vi "Code 0.0.1.vi"() -> ()   [LabVIEW 2017]
uses:
  <vilib>/Instr/_visa.llb/VISA Configure Serial Port (Instr).vi
panel:
  in  "Flash Baudrate":u32(ring)=230400 items=["4800"=4800, "9600"=9600, "19200"=19200, "38400"=38400, "57600"=57600, "115200"=115200, "230400"=230400, "460800"=460800, "921600"=921600]
  in  "cmd Baudrate":u32(ring)=230400 items=["4800"=4800, "9600"=9600, "19200"=19200, "38400"=38400, "57600"=57600, "115200"=115200, "230400"=230400, "460800"=460800, "921600"=921600]
  in  "UUT COM Port":refnum<visa-resource-name>="COM4"
  in  "Next Button":bool
  in  "File Path Control":path
  out "Status":bool
  out "cmd Sent":bool
  out "CheckSumArray":u16[][](array[numeric]) format="%.0x"
  out "CheckSum":bool[][](array[boolean])
  in  "stop 9":bool
  in  "stop 8":bool
  out "CheckSum DataB":u16 format="%.0x"
  out "CheckSum Data":u16 format="%.0x"
  in  "stop 5":bool
  in  "stop 4":bool
  out "Array 3":u16[][](array[numeric]) format="%.0x"
  out "Num of Data packet":i32
  out "Writting Data":bool
  out "Size of Text File":i32
  out "Full Text File":u8[](array[numeric]) format="%.0x"
  out "All bytes in file in HEX U8":u8[](array[numeric]) format="%02x"
  out "Send Header":bool
  out "AutoBaud Success":bool
  out "sumHeader":u16 format="%.0x"
  in  "stop 3":bool
  in  "stop 2":bool
  out "error out":errorcluster
  in  "stop":bool
  out "Autobaud":string
  # "Ver 0.0.1"
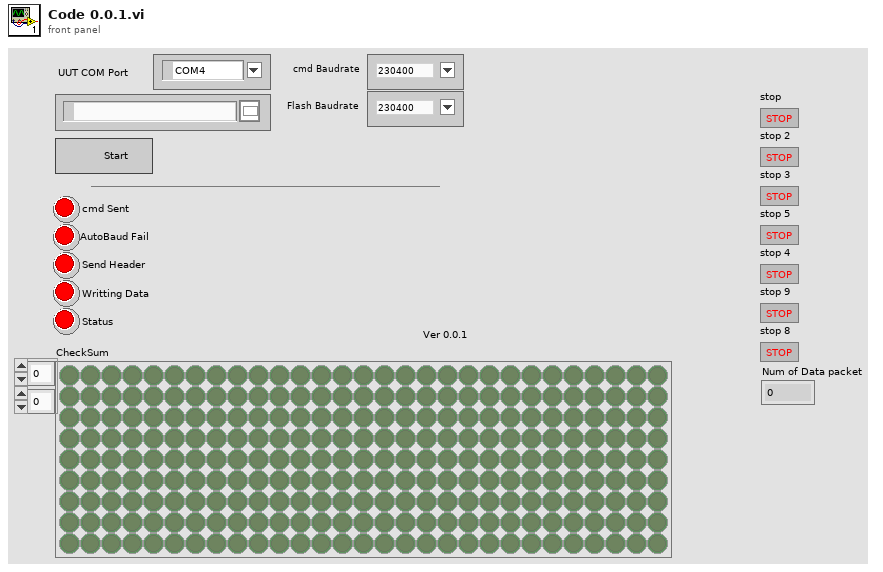
[diagram p1: front panel]
types:
  T1 = enum16{"open", "replace", "create", "open or create", "replace or create", "replace or create with confirmation"}
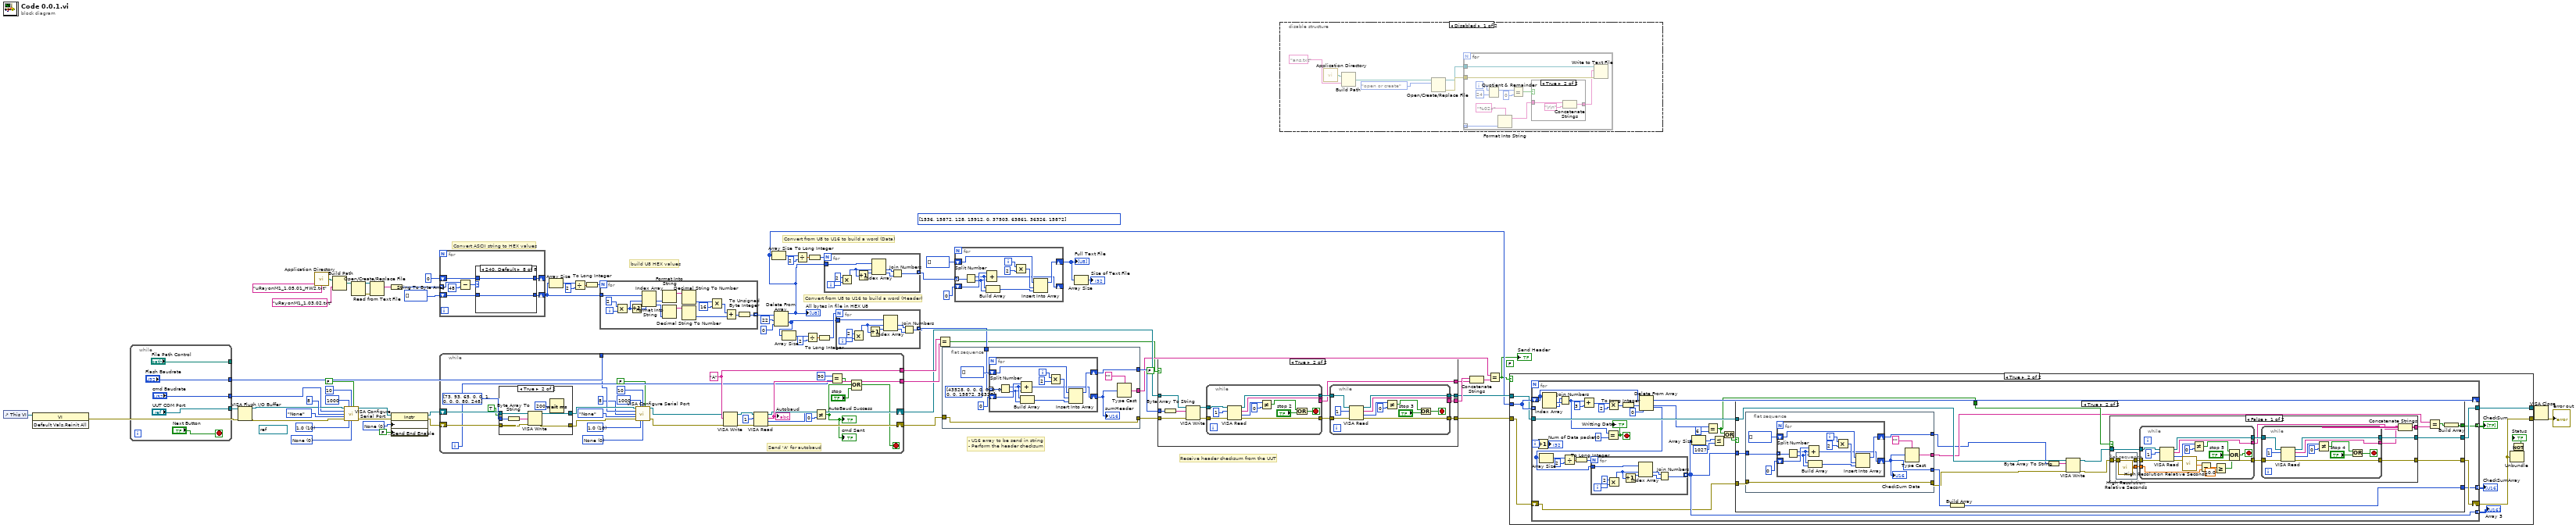
[diagram p0: block diagram]
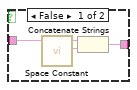
[diagram p3: hidden frame]
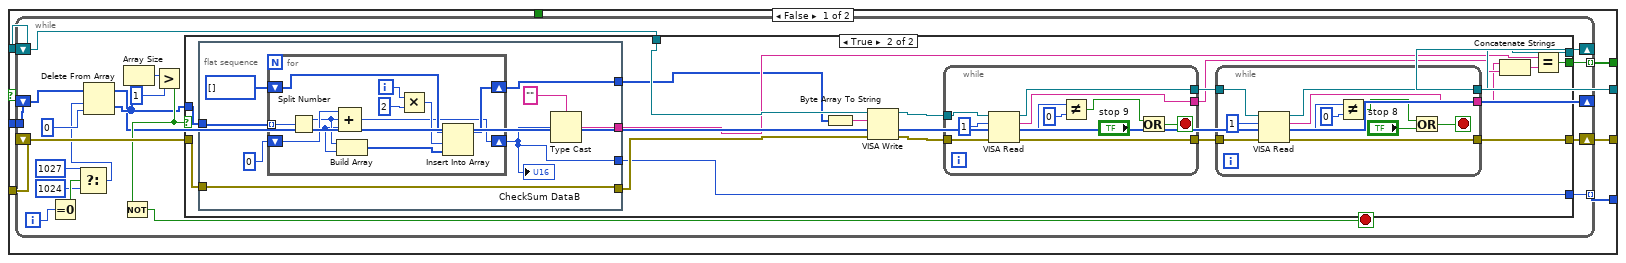
[diagram p6: hidden frame]
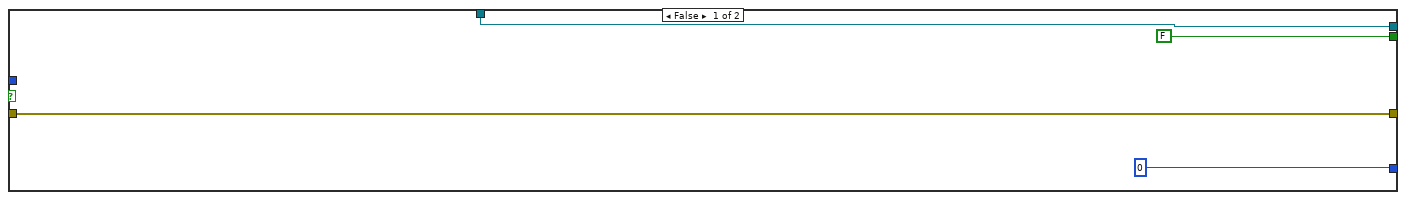
[diagram p7: hidden frame]
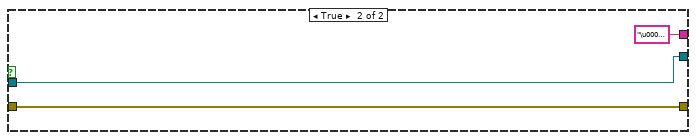
[diagram p8: hidden frame]
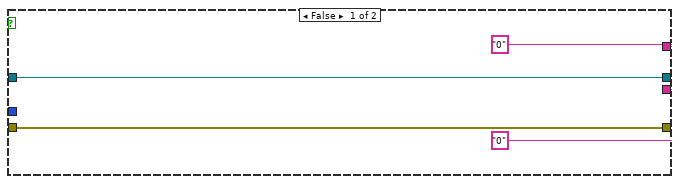
[diagram p9: hidden frame]
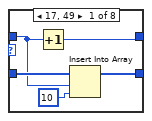
[diagram p10: hidden frame]
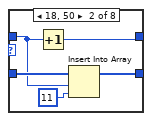
[diagram p11: hidden frame]
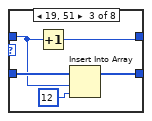
[diagram p12: hidden frame]
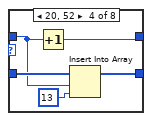
[diagram p13: hidden frame]
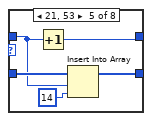
[diagram p14: hidden frame]
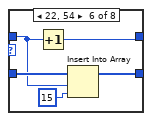
[diagram p15: hidden frame]
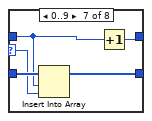
[diagram p16: hidden frame]
diagram:
  (unwired) FALSE
  (unwired) FALSE
  (unwired) u16[] [1536, 15872, 128, 15912, 0, 37503, 63861, 36326, 15872] ("Array 4")
  (unwired) refnum<visa-resource-name> "COM4" ("VISA resource name")
  w32 = u16 0 items=["None", "LastBit", "TermChar", "Break"] ("Serial Settings:Serial End Mode for Writes")
  w36 = u16 0 items=["None", "XON/XOFF", "RTS/CTS", "XON/XOFF & RTS/CTS", "DTR/DSR", "XON/XOFF & DTR/DSR"] ("flow control (0:none)")
  w37 = u16 10 items=["1.0"=10, "1.5"=15, "2.0"=20] ("stop bits (10: 1 bit)")
  (unwired) "uRayonM1_1.05.01_HW2.txt" ("name or relative path")
  # "Receive header checksum from the UUT"
  # "- U16 array to be send in string\n- Perform the header checksum"
  # "Convert from U8 to U16 to build a word (Header)"
  # "build U8 HEX values"
  # "Convert from U8 to U16 to build a word (Data)"
  # "Convert ASCII string to HEX values"
  n1 = control-ref of="This VI"() -> (w8:refnum<vi>)
  n2 = invoke class="VI" method="Default Vals.Reinit All"(reference=w8) -> (error out=w11:errorcluster)  [unwired: 2 in, 2 out]
  n3 = while {
    tunnel: ["UUT COM Port"] -> w4
    tunnel: ["Flash Baudrate"] -> w3
    tunnel: ["cmd Baudrate"] -> w2
    tunnel: ["File Path Control"] -> _
    stop <- "Next Button" stop-if-true
  }
  n4 = VISA Flush I/O Buffer(VISA resource name=w4, error in (no error)=w11) -> (VISA resource name out=w9:refnum<visa-resource-name>, error out=w10:errorcluster)  [unwired: 1 in]
  n5 = call <vilib>:"Application Directory.vi"() -> ("Application Directory"=w63:path)
  n6 = Build Path(base path=w63, name or relative path="uRayonM1_1.03.02.txt") -> (appended path=w1:path)
  n7 = call-poly "VISA Configure Serial Port"("VISA resource name"=w9, "timeout (10sec)"=u32 1000, "termination char\n(0xA = '\\n' = LF)"=u8 10 ("termination char\n(0xA = '\\n' = LF)"), "Enable Termination\nChar (T)"=FALSE ("Enable Termination\nChar (T)"), "baud rate (9600)"=w2, "data bits (8)"=u16 8, "parity (0:none)"=enum16{"None", "Odd", "Even", "Mark", "Space"}."None", "error in (no error)"=w10, "stop bits (10: 1 bit)"=w37, "flow control (0:none)"=w36) -> ("VISA resource name out"=w34:refnum<visa-resource-name>, "error out"=w35:errorcluster)  [unwired: 4 in]
  n8 = Open/Create/Replace File(file path (use dialog)=w1) -> (refnum out=w61:refnum<file>, error out=w62:errorcluster)  [unwired: 5 in, 1 out]
  n9 = Read from Text File(file (use dialog)=w61, error in=w62) -> (text=w59:string)  [unwired: 2 in, 3 out]
  n10 = String To Byte Array(string=w59) -> (unsigned byte array=w60:u8[])
  n11 = property class="Instr"(reference=w34, error in=w35, "Serial Settings:End Mode for Writes"=w32, "Message Based Settings:Send End Enable"=FALSE) -> (reference out=w7:refnum<visa-resource-name>, error out=w6:errorcluster)
  n12 = for {
    tunnel: w60 -> [w82] mode=indexing
    shift-right: [w78] -> w56
    shift-left: u8[] [] -> [w79]
    shift-right: [w77] -> _
    shift-left: 0 ("y") -> [w76]
    n13 = Subtract(x=w82, y=u8 48) -> (x-y=w80:u8)
    n14 = case shown="240, Default" w80 {
      selector: w80 -> [_ _ _ _ _ _ w116 _]
      tunnel: [w85 w90 w96 w100 w105 w110 w115 w119] -> w78
      tunnel: w79 -> [w87 w91 w97 w102 w107 w112 w117 w119]
      tunnel: [w83 w88 w93 w98 w103 w108 w113 w118] -> w77
      tunnel: w76 -> [w84 w89 w94 w99 w104 w109 w114 w118]
      frame 17, 49 {
        n15 = Increment(x=w84) -> (x+1=w83:i32)
        n16 = Insert Into Array(array=w87, index=w84, new element=u8 10) -> (w85:u8[])
      }
      frame 18, 50 {
        n17 = Increment(x=w89) -> (x+1=w88:i32)
        n18 = Insert Into Array(array=w91, index=w89, new element=u8 11) -> (w90:u8[])
      }
      frame 19, 51 {
        n19 = Increment(x=w94) -> (x+1=w93:i32)
        n20 = Insert Into Array(array=w97, index=w94, new element=u8 12) -> (w96:u8[])
      }
      frame 20, 52 {
        n21 = Increment(x=w99) -> (x+1=w98:i32)
        n22 = Insert Into Array(array=w102, index=w99, new element=u8 13) -> (w100:u8[])
      }
      frame 21, 53 {
        n23 = Increment(x=w104) -> (x+1=w103:i32)
        n24 = Insert Into Array(array=w107, index=w104, new element=u8 14) -> (w105:u8[])
      }
      frame 22, 54 {
        n25 = Increment(x=w109) -> (x+1=w108:i32)
        n26 = Insert Into Array(array=w112, index=w109, new element=u8 15) -> (w110:u8[])
      }
      frame 0..9 {
        n27 = Insert Into Array(array=w117, index=w114, new element=w116) -> (w115:u8[])
        n28 = Increment(x=w114) -> (x+1=w113:i32)
      }
      frame 240, Default {
      }
    }
  }
  n29 = while {
    tunnel: [w150] -> w70
    tunnel: [w149] -> w69
    shift-right: [w148] -> w68
    shift-left: w7 -> [w146]
    shift-right: [w147] -> w66
    shift-left: w6 -> [w145]
    tunnel: w3 -> [w127]
    i -> [w133]
    stop <- w136 stop-if-true
    w120 = u16 0 items=["None", "XON/XOFF", "RTS/CTS", "XON/XOFF & RTS/CTS", "DTR/DSR", "XON/XOFF & DTR/DSR"] ("flow control (0:none)")
    w121 = u16 10 items=["1.0"=10, "1.5"=15, "2.0"=20] ("stop bits (10: 1 bit)")
    w149 = "A" ("write buffer")
    # "Send 'A' for autobaud"
    n30 = case shown="True" TRUE {
      tunnel: w146 -> [w152 w159]
      tunnel: w145 -> [w151 w158]
      tunnel: [w152 w157] -> w128
      tunnel: [w151 w156] -> w129
      tunnel: u8[] [73, 93, 65, 0, 0, 1, 0, 0, 0, 80, 248] ("output array") -> [_ w155]
      frame False {
      }
      frame True {
        n31 = Byte Array To String(unsigned byte array=w155) -> (string=w154:string)
        n32 = VISA Write(VISA resource name=w159, write buffer=w154, error in (no error)=w158) -> (VISA resource name out=w157:refnum<visa-resource-name>, error out=w156:errorcluster)  [unwired: 1 out]
        n33 = Wait (ms)(milliseconds to wait=u32 200) -> ()  [unwired: 1 out]
      }
    }
    n34 = call-poly "VISA Configure Serial Port"("VISA resource name"=w128, "timeout (10sec)"=u32 1000, "termination char\n(0xA = '\\n' = LF)"=u8 10 ("termination char\n(0xA = '\\n' = LF)"), "Enable Termination\nChar (T)"=FALSE ("Enable Termination\nChar (T)"), "baud rate (9600)"=w127, "data bits (8)"=u16 8, "parity (0:none)"=enum16{"None", "Odd", "Even", "Mark", "Space"}."None", "error in (no error)"=w129, "stop bits (10: 1 bit)"=w121, "flow control (0:none)"=w120) -> ("VISA resource name out"=w130:refnum<visa-resource-name>, "error out"=w131:errorcluster)  [unwired: 4 in]
    n35 = VISA Write(VISA resource name=w130, write buffer=w149, error in (no error)=w131) -> (VISA resource name out=w139:refnum<visa-resource-name>, error out=w138:errorcluster)  [unwired: 1 out]
    n36 = VISA Read(VISA resource name=w139, byte count=u32 1, error in (no error)=w138) -> (VISA resource name out=w148:refnum<visa-resource-name>, read buffer=w150:string, return count=w141:u32, error out=w147:errorcluster)
    "Autobaud" <- w150
    n37 = Not Equal?(x=w141, y=u32 0) -> (x != y?=w132:bool)
    "AutoBaud Success" <- w132
    "cmd Sent" <- w132
    n38 = Equal?(x=90, y=w133) -> (x = y?=w134:bool)
    n39 = Compound Arithmetic op=OR(w134, w132, "stop") -> (w136:bool)
  }
  n40 = Array Size(array=w56) -> (size(s)=w55:i32)
  n41 = Divide(x=w55, y=2) -> (x/y=w53:dbl)
  n42 = To Long Integer(number=w53) -> (32bit integer=w52:i32)
  n43 = for {
    N: w52 -> [_]
    tunnel: w56 -> [w174]
    tunnel: [w160] -> w51 mode=indexing
    i -> [w173]
    n44 = Multiply(x=2, y=w173) -> (x*y=w171:i32)
    n45 = Increment(x=w171) -> (x+1=w170:i32)
    n46 = Index Array(array=w174, index #1=w171, index #2=w170) -> (element #1=w163:u8, element #2=w162:u8)
    n47 = Format Into String(w163) -> (resulting string=w164:string)  [unwired: 3 in, 1 out]
    n48 = Format Into String(w162) -> (resulting string=w169:string)  [unwired: 3 in, 1 out]
    n49 = Decimal String To Number(string=w164) -> (number=w165:i32)  [unwired: 2 in, 1 out]
    n50 = Decimal String To Number(string=w169) -> (number=w168:i32)  [unwired: 2 in, 1 out]
    n51 = Multiply(x=w165, y=16) -> (x*y=w167:i32)
    n52 = Add(x=w167, y=w168) -> (x+y=w161:i32)
    n53 = To Unsigned Byte Integer(number=w161) -> (unsigned 8bit integer=w160:u8)
  }
  n54 = Delete From Array(array=w51, length=22, index=0) -> (deleted portion=w22:u8[], array with subset deleted=w14:u8[])
  "All bytes in file in HEX U8" <- w14
  n55 = Array Size(array=w14) -> (size(s)=w28:i32)
  n56 = Array Size(array=w22) -> (size(s)=w27:i32)
  n57 = Divide(x=w28, y=2) -> (x/y=w30:dbl)
  n58 = Divide(x=w27, y=2) -> (x/y=w25:dbl)
  n59 = To Long Integer(number=w30) -> (32bit integer=w23:i32)
  n60 = To Long Integer(number=w25) -> (32bit integer=w24:i32)
  n61 = for {
    N: w23 -> [_]
    tunnel: w14 -> [w179]
    tunnel: [w175] -> w15 mode=indexing
    i -> [w178]
    n62 = Multiply(x=2, y=w178) -> (x*y=w181:i32)
    n63 = Increment(x=w181) -> (x+1=w182:i32)
    n64 = Index Array(array=w179, index #1=w181, index #2=w182) -> (element #1=w177:u8, element #2=w176:u8)
    n65 = Join Numbers(hi=w177, lo=w176) -> ((hi.lo)=w175:u16)
  }
  n66 = for {
    N: w24 -> [_]
    tunnel: w22 -> [w187]
    tunnel: [w183] -> w21 mode=indexing
    i -> [w186]
    n67 = Multiply(x=2, y=w186) -> (x*y=w189:i32)
    n68 = Increment(x=w189) -> (x+1=w190:i32)
    n69 = Index Array(array=w187, index #1=w189, index #2=w190) -> (element #1=w185:u8, element #2=w184:u8)
    n70 = Join Numbers(hi=w185, lo=w184) -> ((hi.lo)=w183:u16)
  }
  n71 = Equal?(x=w69, y=w70) -> (x = y?=w12:bool)
  n72 = flat-sequence {
    tunnel: w66 -> [w191]
    tunnel: [w196] -> w65
    tunnel: [w193] -> w64
    tunnel: w21 -> [w192]
    tunnel: [w191] -> w20
    frame #0 {
      (unwired) u16[] [43528, 0, 0, 0, 0, 0, 0, 0, 0, 15872, 36326]
      n73 = for {
        tunnel: w192 -> [w209] mode=indexing
        shift-right: [w204] -> w196
        shift-left: u8[] [] -> [w203]
        shift-right: [w201] -> w195
        shift-left: u16 0 -> [w202]
        i -> [w208]
        n74 = Split Number(x=w209) -> (hi(x)=w200:u8, lo(x)=w199:u8)
        n75 = Build Array(w200, w199) -> (w206:u8[])
        n76 = Compound Arithmetic op=ADD(w202, w200, w199) -> (w201:u16)
        n77 = Multiply(x=w208, y=2) -> (x*y=w205:i32)
        n78 = Insert Into Array(array=w203, index=w205, new element=w206) -> (w204:u8[])
      }
      "sumHeader" <- w195
      n79 = Type Cast(type="", x=w195) -> (*(type *) &x=w193:string)
    }
  }
  n80 = for {
    tunnel: w15 -> [w220] mode=indexing
    shift-right: [w215] -> w17
    shift-left: u8[] [] -> [w214]
    shift-right: [w212] -> _
    shift-left: u16 0 -> [w213]
    i -> [w219]
    n81 = Split Number(x=w220) -> (hi(x)=w211:u8, lo(x)=w210:u8)
    n82 = Build Array(w211, w210) -> (w217:u8[])
    n83 = Compound Arithmetic op=ADD(w213, w211, w210) -> (w212:u16)
    n84 = Multiply(x=w219, y=2) -> (x*y=w216:i32)
    n85 = Insert Into Array(array=w214, index=w216, new element=w217) -> (w215:u8[])
  }
  "Full Text File" <- w17
  n86 = Array Size(array=w17) -> (size(s)=→"Size of Text File":i32)
  n87 = case shown="True" w12 {
    tunnel: w20 -> [w223 w232]
    tunnel: w68 -> [w224 w231]
    tunnel: [w223 w230] -> w42
    tunnel: [w224 w229] -> w43
    tunnel: w65 -> [_ w228]
    tunnel: ["0" ("read buffer") w227] -> w46
    tunnel: ["0" ("read buffer") w226] -> w45
    frame False {
    }
    frame True {
      n88 = Byte Array To String(unsigned byte array=w228) -> (string=w225:string)
      n89 = VISA Write(VISA resource name=w231, write buffer=w225, error in (no error)=w232) -> (VISA resource name out=w234:refnum<visa-resource-name>, error out=w233:errorcluster)  [unwired: 1 out]
      n90 = while {
        tunnel: w234 -> [w255]
        tunnel: [w256] -> w235
        tunnel: w233 -> [w254]
        tunnel: [w257] -> w236
        tunnel: [w248] -> w226
        stop <- w250 stop-if-true
        n91 = VISA Read(VISA resource name=w255, byte count=u32 1, error in (no error)=w254) -> (VISA resource name out=w256:refnum<visa-resource-name>, read buffer=w248:string, return count=w249:u32, error out=w257:errorcluster)
        n92 = Not Equal?(x=w249, y=u32 0) -> (x != y?=w252:bool)
        n93 = Or(x=w252, y="stop 2") -> (x .or. y?=w250:bool)
      }
      n94 = while {
        tunnel: w235 -> [w246]
        tunnel: [w243] -> w229
        tunnel: w236 -> [w247]
        tunnel: [w244] -> w230
        tunnel: [w237] -> w227
        stop <- w238 stop-if-true
        n95 = VISA Read(VISA resource name=w246, byte count=u32 1, error in (no error)=w247) -> (VISA resource name out=w243:refnum<visa-resource-name>, read buffer=w237:string, return count=w239:u32, error out=w244:errorcluster)
        n96 = Not Equal?(x=w239, y=u32 0) -> (x != y?=w242:bool)
        n97 = Or(x=w242, y="stop 3") -> (x .or. y?=w238:bool)
      }
    }
  }
  n98 = disable-structure shown="Disabled" {
    frame Disabled {
      n99 = call <vilib>:"Application Directory.vi"() -> ("Application Directory"=w263:path)
      n100 = Build Path(base path=w263, name or relative path="ans.txt") -> (appended path=w262:path)
      n101 = Open/Create/Replace File(file path (use dialog)=w262, operation (0:open)=T1."open or create") -> (refnum out=w259:refnum<file>, error out=w260:errorcluster)  [unwired: 4 in, 1 out]
      n102 = for {
        tunnel: _ -> [w275] mode=indexing
        tunnel: w260 -> [w273]
        tunnel: w259 -> [w272]
        i -> [w268]
        n103 = Quotient & Remainder(x=w268, y=24 ("x")) -> (x-y*floor(x/y)=w266:i32)  [unwired: 1 out]
        n104 = Format Into String(format string="%02x", w275) -> (resulting string=w271:string)  [unwired: 2 in, 1 out]
        n105 = Equal?(x=w266, y=0) -> (x = y?=w269:bool)
        n106 = case shown="True" w269 {
          tunnel: w271 -> [w278 w281]
          tunnel: [w277 w280] -> w270
          frame False {
            n107 = call <vilib>:"Space Constant.vi"() -> ("String"=w276:string)
            n108 = Concatenate Strings(w278, w276) -> (w277:string)
          }
          frame True {
            n109 = Concatenate Strings(w281, "\r\n") -> (w280:string)
          }
        }
        n110 = Write to Text File(file (use dialog)=w272, text=w270, error in=w273) -> ()  [unwired: 1 in, 3 out]
      }
    }
    frame Enabled {
    }
  }
  n111 = Concatenate Strings(w46, w45) -> (w44:string)
  n112 = Equal?(x=w64, y=w44) -> (x = y?=w13:bool)
  "Send Header" <- w13
  n113 = case shown="True" w13 {
    tunnel: w43 -> [w283 w291]
    tunnel: w42 -> [w282 w287]
    tunnel: [w283 w290] -> w48
    tunnel: [w282 w286] -> w47
    tunnel: w14 -> [_ w292]
    frame False {
    }
    frame True {
      n114 = for {
        shift-right: [w315] -> _
        shift-left: w292 -> [w326]
        tunnel: w292 -> [_] mode=indexing
        tunnel: [w308] -> w293 mode=indexing
        tunnel: w291 -> [w307]
        tunnel: [w303] -> w290
        tunnel: [w301] -> w289 mode=indexing
        tunnel: [w300] -> w288 mode=indexing
        shift-right: [w302] -> w286
        shift-left: w287 -> [w294]
        i -> [w316]
        stop <- w319 stop-if-true
        n115 = Increment(x=w316) -> (x+1=→"Num of Data packet":i32)
        n116 = Index Array(array=w326) -> (element #1=w325:u8, element #2=w324:u8)  [unwired: 2 in]
        n117 = Join Numbers(hi=w324, lo=w325) -> ((hi.lo)=w296:u16)
        n118 = Add(x=w296, y=u32 3) -> (x+y=w322:u32)
        n119 = Equal?(x=w296, y=u16 0) -> (x = y?=w319:bool)
        "Writting Data" <- w319
        n120 = Multiply(x=w322, y=u32 2) -> (x*y=w320:u32)
        n121 = To Long Integer(number=w320) -> (32bit integer=w297:i32)
        n122 = Delete From Array(array=w326, length=w297, index=0) -> (deleted portion=w298:u8[], array with subset deleted=w315:u8[])
        n123 = Array Size(array=w298) -> (size(s)=w312:i32)
        n124 = Divide(x=w312, y=2) -> (x/y=w314:dbl)
        n125 = To Long Integer(number=w314) -> (32bit integer=w311:i32)
        n126 = for {
          N: w311 -> [_]
          tunnel: w298 -> [w499]
          tunnel: [w495] -> w308 mode=indexing
          i -> [w498]
          n127 = Multiply(x=2, y=w498) -> (x*y=w501:i32)
          n128 = Increment(x=w501) -> (x+1=w502:i32)
          n129 = Index Array(array=w499, index #1=w501, index #2=w502) -> (element #1=w497:u8, element #2=w496:u8)
          n130 = Join Numbers(hi=w497, lo=w496) -> ((hi.lo)=w495:u16)
        }
        n131 = Array Size(array=w308) -> (size(s)=w310:i32)
        n132 = Equal?(x=w297, y=6) -> (x = y?=w295:bool)
        n133 = Less Or Equal?(x=w310, y=1027) -> (x <= y?=w305:bool)
        n134 = Or(x=w295, y=w305) -> (x .or. y?=w304:bool)
        n135 = case shown="True" w304 {
          tunnel: w294 -> [w330 w429]
          tunnel: w307 -> [w333 w420]
          tunnel: [w332 w432] -> w302
          tunnel: [w331 w431] -> w303
          tunnel: w308 -> [w328 w430]
          tunnel: [w329 w426] -> w301
          tunnel: [w327 w424] -> w300
          tunnel: w295 -> [_ w423]
          frame False {
            n136 = while {
              tunnel: w328 -> [_]
              tunnel: [w348] -> w329 mode=indexing
              shift-right: [w350] -> w331
              shift-left: w333 -> [w352]
              shift-right: [w351] -> w332
              shift-left: w330 -> [w349]
              shift-right: [w340] -> _
              shift-left: w328 -> [w347]
              tunnel: [w339] -> w327 mode=indexing
              i -> [w338]
              stop <- w342 stop-if-true
              n137 = Equal To 0?(x=w338) -> (x = 0?=w337:bool)
              n138 = Select(t=1027 ("length"), s=w337, f=1024 ("length")) -> (s? t:f=w334:i32)
              n139 = Delete From Array(array=w347, length=w334, index=0) -> (deleted portion=w341:u16[], array with subset deleted=w340:u16[])
              n140 = Array Size(array=w341) -> (size(s)=w345:i32)
              n141 = Greater?(x=w345, y=1) -> (0:w343:bool)
              n142 = Not(x=w343) -> (.not. x?=w342:bool)
              n143 = case shown="True" w343 {
                tunnel: w352 -> [w354 w370]
                tunnel: [w356 w369] -> w351
                tunnel: [w354 w368] -> w350
                tunnel: w349 -> [w356 w366]
                tunnel: [FALSE w361] -> w348
                tunnel: w341 -> [_ w360]
                tunnel: [u16 0 ("Numeric") w359] -> w339
                frame False {
                }
                frame True {
                  n144 = flat-sequence {
                    tunnel: w366 -> [w376]
                    tunnel: [w380] -> w357
                    tunnel: [w378] -> w362
                    tunnel: w360 -> [w377]
                    tunnel: [w376] -> w367
                    tunnel: [w375] -> w359
                    frame #0 {
                      n145 = for {
                        tunnel: w377 -> [w393] mode=indexing
                        shift-right: [w388] -> w380
                        shift-left: u8[] [] -> [w387]
                        shift-right: [w385] -> w375
                        shift-left: u16 0 -> [w386]
                        i -> [w392]
                        n146 = Split Number(x=w393) -> (hi(x)=w384:u8, lo(x)=w383:u8)
                        n147 = Build Array(w384, w383) -> (w390:u8[])
                        n148 = Compound Arithmetic op=ADD(w386, w384, w383) -> (w385:u16)
                        n149 = Multiply(x=w392, y=2) -> (x*y=w389:i32)
                        n150 = Insert Into Array(array=w387, index=w389, new element=w390) -> (w388:u8[])
                      }
                      "CheckSum DataB" <- w375
                      n151 = Type Cast(type="", x=w375) -> (*(type *) &x=w378:string)
                    }
                  }
                  n152 = Byte Array To String(unsigned byte array=w357) -> (string=w358:string)
                  n153 = VISA Write(VISA resource name=w370, write buffer=w358, error in (no error)=w367) -> (VISA resource name out=w372:refnum<visa-resource-name>, error out=w371:errorcluster)  [unwired: 1 out]
                  n154 = while {
                    tunnel: w372 -> [w412]
                    tunnel: [w413] -> w373
                    tunnel: w371 -> [w411]
                    tunnel: [w414] -> w374
                    tunnel: [w405] -> w365
                    stop <- w407 stop-if-true
                    n155 = VISA Read(VISA resource name=w412, byte count=u32 1, error in (no error)=w411) -> (VISA resource name out=w413:refnum<visa-resource-name>, read buffer=w405:string, return count=w406:u32, error out=w414:errorcluster)
                    n156 = Not Equal?(x=w406, y=u32 0) -> (x != y?=w409:bool)
                    n157 = Or(x=w409, y="stop 9") -> (x .or. y?=w407:bool)
                  }
                  n158 = while {
                    tunnel: w373 -> [w403]
                    tunnel: [w400] -> w368
                    tunnel: w374 -> [w404]
                    tunnel: [w401] -> w369
                    tunnel: [w394] -> w364
                    stop <- w395 stop-if-true
                    n159 = VISA Read(VISA resource name=w403, byte count=u32 1, error in (no error)=w404) -> (VISA resource name out=w400:refnum<visa-resource-name>, read buffer=w394:string, return count=w396:u32, error out=w401:errorcluster)
                    n160 = Not Equal?(x=w396, y=u32 0) -> (x != y?=w399:bool)
                    n161 = Or(x=w399, y="stop 8") -> (x .or. y?=w395:bool)
                  }
                  n162 = Concatenate Strings(w364, w365) -> (w363:string)
                  n163 = Equal?(x=w362, y=w363) -> (x = y?=w361:bool)
                }
              }
            }
          }
          frame True {
            n164 = flat-sequence {
              tunnel: w429 -> [w477]
              tunnel: [w481] -> w416
              tunnel: [w479] -> w418
              tunnel: w430 -> [w478]
              tunnel: [w477] -> w419
              tunnel: [w476] -> w425
              frame #0 {
                n165 = for {
                  tunnel: w478 -> [w494] mode=indexing
                  shift-right: [w489] -> w481
                  shift-left: u8[] [] -> [w488]
                  shift-right: [w486] -> w476
                  shift-left: u16 0 -> [w487]
                  i -> [w493]
                  n166 = Split Number(x=w494) -> (hi(x)=w485:u8, lo(x)=w484:u8)
                  n167 = Build Array(w485, w484) -> (w491:u8[])
                  n168 = Compound Arithmetic op=ADD(w487, w485, w484) -> (w486:u16)
                  n169 = Multiply(x=w493, y=2) -> (x*y=w490:i32)
                  n170 = Insert Into Array(array=w488, index=w490, new element=w491) -> (w489:u8[])
                }
                "CheckSum Data" <- w476
                n171 = Type Cast(type="", x=w476) -> (*(type *) &x=w479:string)
              }
            }
            n172 = Build Array(w425) -> (w424:u16[])
            n173 = Byte Array To String(unsigned byte array=w416) -> (string=w417:string)
            n174 = VISA Write(VISA resource name=w420, write buffer=w417, error in (no error)=w419) -> (VISA resource name out=w421:refnum<visa-resource-name>, error out=w422:errorcluster)  [unwired: 1 out]
            n175 = case shown="False" w423 {
              tunnel: w421 -> [w441 w474]
              tunnel: w422 -> [w434 w473]
              tunnel: [w440 w473] -> w432
              tunnel: [w439 w474] -> w431
              tunnel: [w436 "\u0000\u0000"] -> w428
              frame False {
                n176 = flat-sequence {
                  tunnel: [w445] -> w435
                  tunnel: w434 -> [w444]
                  tunnel: [w444] -> w433
                  frame #0 {
                    n177 = call <vilib>:"High Resolution Relative Seconds.vi"() -> ("relative seconds"=w445:dbl)
                  }
                }
                n178 = while {
                  tunnel: w441 -> [w469]
                  tunnel: [w470] -> w442
                  tunnel: w433 -> [w468]
                  tunnel: [w471] -> w443
                  tunnel: [w462] -> w438
                  tunnel: w435 -> [w460]
                  stop <- w464 stop-if-true
                  n179 = VISA Read(VISA resource name=w469, byte count=u32 1, error in (no error)=w468) -> (VISA resource name out=w470:refnum<visa-resource-name>, read buffer=w462:string, return count=w463:u32, error out=w471:errorcluster)
                  n180 = call <vilib>:"High Resolution Relative Seconds.vi"() -> ("relative seconds"=w461:dbl)
                  n181 = Not Equal?(x=w463, y=u32 0) -> (x != y?=w466:bool)
                  n182 = Subtract(x=w461, y=w460) -> (x-y=w459:dbl)
                  n183 = Greater Or Equal?(x=w459, y=10.0) -> (x >= y?=w457:bool)
                  n184 = Compound Arithmetic op=OR(w466, "stop 5", w457) -> (w464:bool)
                }
                n185 = while {
                  tunnel: w442 -> [w455]
                  tunnel: [w452] -> w439
                  tunnel: w443 -> [w456]
                  tunnel: [w453] -> w440
                  tunnel: [w446] -> w437
                  stop <- w447 stop-if-true
                  n186 = VISA Read(VISA resource name=w455, byte count=u32 1, error in (no error)=w456) -> (VISA resource name out=w452:refnum<visa-resource-name>, read buffer=w446:string, return count=w448:u32, error out=w453:errorcluster)
                  n187 = Not Equal?(x=w448, y=u32 0) -> (x != y?=w451:bool)
                  n188 = Or(x=w451, y="stop 4") -> (x .or. y?=w447:bool)
                }
                n189 = Concatenate Strings(w437, w438) -> (w436:string)
              }
              frame True {
              }
            }
            n190 = Equal?(x=w418, y=w428) -> (x = y?=w427:bool)
            n191 = Build Array(w427) -> (w426:bool[])
          }
        }
      }
      "Array 3" <- w293
      "CheckSum" <- w289
      "CheckSumArray" <- w288
      n192 = Unbundle(w286) -> ("status"=w285:bool)  [unwired: 2 out]
      n193 = Not(x=w285) -> (.not. x?=→"Status":bool)
    }
  }
  n194 = VISA Close(VISA resource name=w48, error in (no error)=w47) -> (error out=→"error out":errorcluster)
